vi "IsParent.vi"(8 "error in (no error)":errorcluster, 10 "index":i32, 11 "menu in":refnum<class "menu.lvclass">) -> (0 "error out":errorcluster, 2 "parent?":bool, 3 "menu out":refnum<class "menu.lvclass">)   [LabVIEW 2009, in "menu.lvclass"]
uses:
  menu.lvclass
  menu.lvclass/menu.ctl
  Menu Item/menu item.lvclass
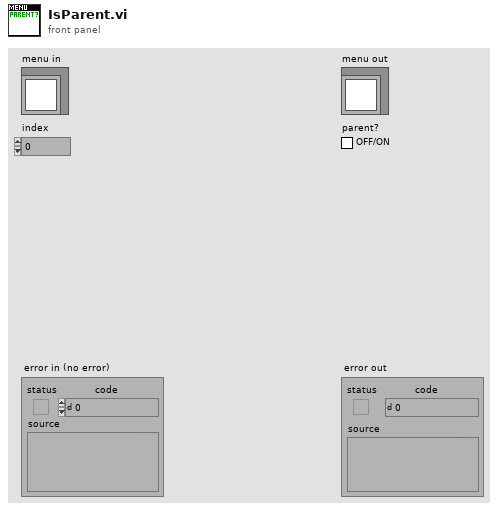
[diagram p1: front panel]
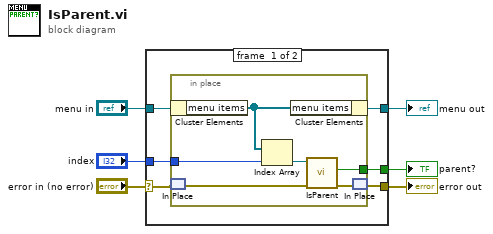
[diagram p0: block diagram]
diagram:
  n1 = case shown="No Error" "error in (no error)" {
    selector: "error in (no error)" -> [w8 w20]
    tunnel: [w7 w20] -> w3
    tunnel: [w11 w19] -> w5
    tunnel: "menu in" -> [w12 w19]
    tunnel: "index" -> [w10 _]
    tunnel: [w9 _] -> w1
    frame #0 {
      n2 = in-place {
        in-place-border: w10 -> [w17]
        in-place-border: [w15] -> w9
        n3 = in-place-cluster #1(w12) -> ("menu items"=w18:refnum<class "menu item.lvclass">[])
        n4 = in-place-match #2(w8) -> (w14:errorcluster)
        n5 = Index Array(array=w18, index=w17) -> (element=w16:refnum<class "menu item.lvclass">)
        n6 = in-place-cluster #1("menu items"=w18) -> (w11:refnum<class "menu.lvclass">)
        n7 = call-dynamic "IsParent.vi"("error in (no error)"=w14, "menu item in"=w16) -> ("error out"=w13:errorcluster, "parent?"=w15:bool)  [unwired: 7 in, 1 out]
        n8 = in-place-match #2(w13) -> (w7:errorcluster)
      }
    }
    frame #1 {
    }
  }
  "menu out" <- w5
  "error out" <- w3
  "parent?" <- w1
